vi "Agilent PWM Format Model String.vi"(1 "Model":string) -> (0 "Model":T1)   [LabVIEW 2011]
uses:
  TypeDefs/Agilent PWM Model.ctl
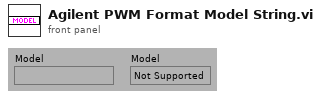
[diagram p1: front panel]
types:
  T1 = typedef "Agilent PWM Model.ctl" = enum16{"Not Supported", "E4418X", "E4419X", "U2000X"}
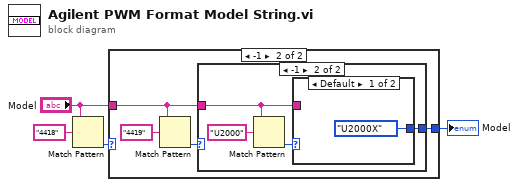
[diagram p0: block diagram]
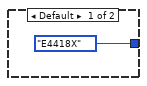
[diagram p2: hidden frame]
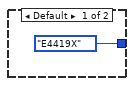
[diagram p3: hidden frame]
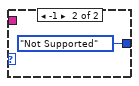
[diagram p4: hidden frame]
diagram:
  n1 = Match Pattern(string="Model", regular expression="4418") -> (offset past match=w2:i32)  [unwired: 4 out]
  n2 = case shown="-1" w2 {
    tunnel: [Agilent_PWM_Model."E4418X" ("Model") w9] -> w1
    tunnel: "Model" -> [_ w7]
    frame Default {
    }
    frame -1 {
      n3 = Match Pattern(string=w7, regular expression="4419") -> (offset past match=w6:i32)  [unwired: 4 out]
      n4 = case shown="-1" w6 {
        tunnel: [Agilent_PWM_Model."E4419X" ("Model") w14] -> w9
        tunnel: w7 -> [_ w11]
        frame Default {
        }
        frame -1 {
          n5 = Match Pattern(string=w11, regular expression="U2000") -> (offset past match=w12:i32)  [unwired: 4 out]
          n6 = case shown="Default" w12 {
            tunnel: w11 -> [_ _]
            tunnel: [Agilent_PWM_Model."U2000X" ("Model") Agilent_PWM_Model."Not Supported" ("Model")] -> w14
            frame Default {
            }
            frame -1 {
            }
          }
        }
      }
    }
  }
  "Model" <- w1
